vi "Ball Movement Graph with Air Resistance.vi"(0 "X Velocity Initial":dbl, 1 "Y Velocity Initial":dbl, 2 "Initial Angular Velocity":dbl, 3 "X Coordinate Initial":dbl, 4 "Y Coordinate Initial":dbl, 5 "Delta Time":dbl, 7 "milliseconds to wait":u32) -> (10 "Cross-Sectional Area":dbl, 12 "Drag Coefficient":dbl, 14 "Table":string[][](table), 15 "X of Y max":dbl, 16 "Y Max":dbl)   [LabVIEW 2013]
panel:
  out "Loop Count":i32
  out "Y Coordinate":dbl
  out "X Coordinate":dbl
  out "Angular Velocity":dbl
  out "Time":dbl
  out "Y Velocity":dbl
  out "X Velocity":dbl
  out "X Acceleration":dbl
  out "Y Acceleration":dbl
  # "This is in SI"
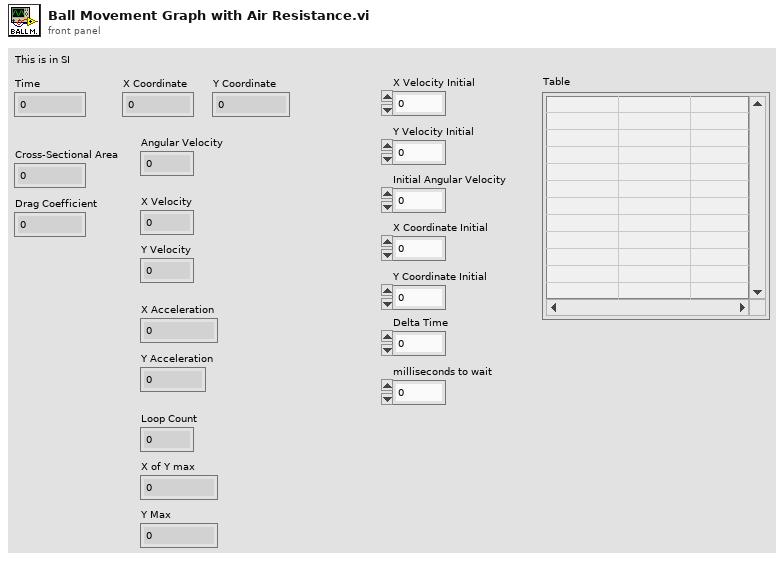
[diagram p1: front panel]
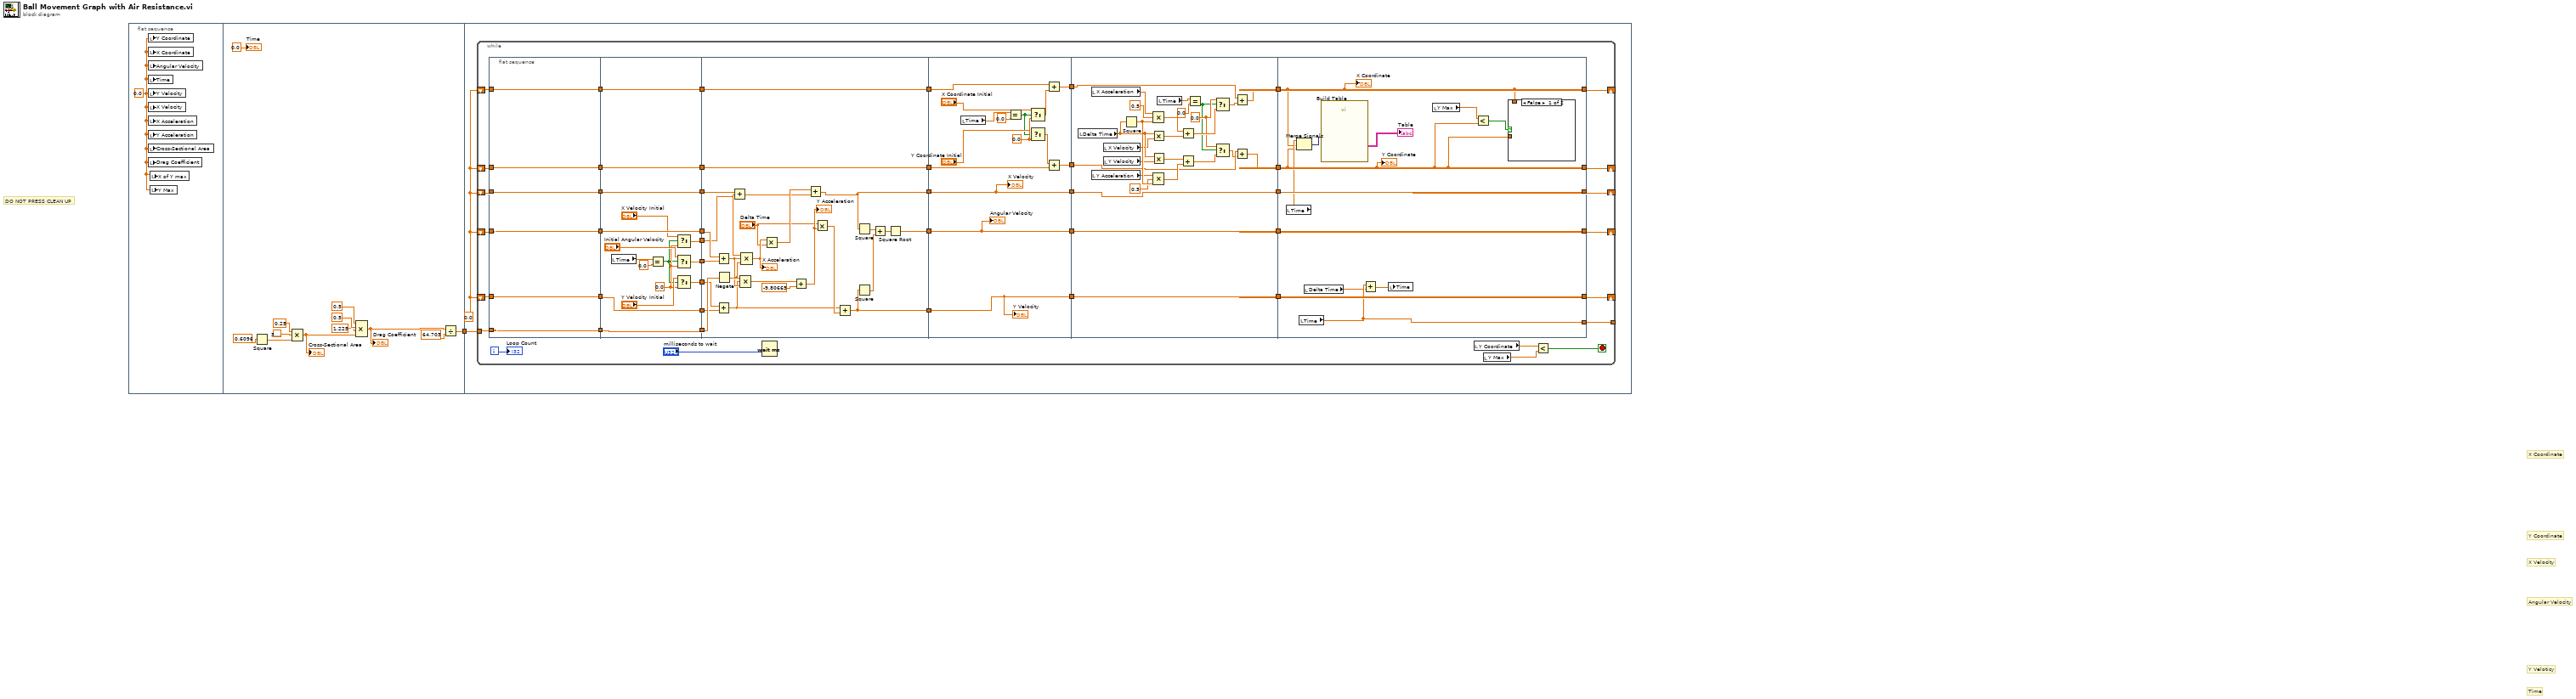
[diagram p0: block diagram]
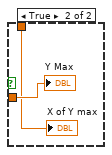
[diagram p2: hidden frame]
diagram:
  # "DO NOT PRESS CLEAN UP"
  # "Time"
  # "X Coordinate"
  # "Y Coordinate"
  # "Angular Velocity"
  # "X Velocity"
  # "Y Veloticy"
  n1 = flat-sequence {
    tunnel: [w6] -> w1
    tunnel: w1 -> [w16]
    frame #0 {
      w2 = 0.0
      n2 = local write "Y Coordinate"(w2) -> ()
      n3 = local write "X Coordinate"(w2) -> ()
      n4 = local write "Angular Velocity"(w2) -> ()
      n5 = local write "Time"(w2) -> ()
      n6 = local write "Y Velocity"(w2) -> ()
      n7 = local write "X Velocity"(w2) -> ()
      n8 = local write "X Acceleration"(w2) -> ()
      n9 = local write "Y Acceleration"(w2) -> ()
      n10 = local write "Cross-Sectional Area"(w2) -> ()
      n11 = local write "Drag Coefficient"(w2) -> ()
      n12 = local write "X of Y max"(w2) -> ()
      n13 = local write "Y Max"(w2) -> ()
    }
    frame #1 {
      n14 = Square(x=0.6096) -> (x^2=w4:dbl)
      n15 = Compound Arithmetic op=MULTIPLY(0.25 ("value"), 3.141592653589793, w4) -> (w3:dbl)
      "Cross-Sectional Area" <- w3
      n16 = Compound Arithmetic op=MULTIPLY(0.5 ("value"), 0.5 ("value"), 1.225 ("value"), w3) -> (w8:dbl)
      "Drag Coefficient" <- w8
      n17 = Divide(x=w8, y=64.703 ("x")) -> (x/y=w6:dbl)
      "Time" <- 0.0 ("Time")
    }
    frame #2 {
      w15 = 0.0
      n18 = while {
        tunnel: w16 -> [w57]
        shift-right: [w49] -> _
        shift-left: w15 -> [w22]
        shift-right: [w50] -> _
        shift-left: w15 -> [w58]
        shift-right: [w51] -> _
        shift-left: w15 -> [w19]
        shift-right: [w26] -> _
        shift-left: w15 -> [w20]
        shift-right: [w25] -> _
        shift-left: w15 -> [w21]
        tunnel: [w24] -> _
        i -> [w23]
        stop <- w27 stop-if-true
        n19 = flat-sequence {
          tunnel: w21 -> [w66]
          tunnel: w20 -> [w65]
          tunnel: w22 -> [w64]
          tunnel: w19 -> [w67]
          tunnel: w58 -> [w68]
          tunnel: w57 -> [w69]
          tunnel: [w69] -> w34
          tunnel: [w68] -> w33
          tunnel: [w67] -> w32
          tunnel: [w64] -> w31
          tunnel: [w65] -> w30
          tunnel: [w66] -> w29
          tunnel: [w85] -> w43
          tunnel: [w84] -> w42
          tunnel: [w70] -> w41
          tunnel: [w83] -> w40
          tunnel: [w82] -> w39
          tunnel: [w81] -> w38
          tunnel: [w80] -> w37
          tunnel: [w79] -> w36
          tunnel: [w78] -> w35
          tunnel: w34 -> [w85]
          tunnel: w33 -> [w84]
          tunnel: w32 -> [w70]
          tunnel: w31 -> [w83]
          tunnel: w30 -> [w82]
          tunnel: w29 -> [w81]
          tunnel: [w100] -> w63
          tunnel: [w110] -> w60
          tunnel: [w92] -> w56
          tunnel: [w91] -> w55
          tunnel: [w90] -> w52
          tunnel: w43 -> [w111]
          tunnel: w42 -> [w87]
          tunnel: w41 -> [w101]
          tunnel: w40 -> [w93]
          tunnel: w39 -> [w91]
          tunnel: w38 -> [w90]
          tunnel: w37 -> [w89]
          tunnel: w36 -> [w86]
          tunnel: w35 -> [w88]
          tunnel: w63 -> [w114]
          tunnel: [w114] -> w62
          tunnel: [w112] -> w61
          tunnel: w60 -> [w113]
          tunnel: [w113] -> w59
          tunnel: w56 -> [w112]
          tunnel: w55 -> [w115]
          tunnel: [w120] -> w54
          tunnel: [w119] -> w53
          tunnel: w52 -> [w116]
          tunnel: w62 -> [w153]
          tunnel: w61 -> [w151]
          tunnel: w59 -> [w152]
          tunnel: w54 -> [w140]
          tunnel: w53 -> [w137]
          tunnel: [w153] -> w48
          tunnel: [w151] -> w47
          tunnel: [w152] -> w46
          tunnel: [w139] -> w45
          tunnel: [w138] -> w44
          tunnel: [w156] -> w25
          tunnel: [w154] -> w26
          tunnel: [w163] -> w50
          tunnel: [w161] -> w49
          tunnel: [w162] -> w51
          tunnel: w48 -> [w162]
          tunnel: w47 -> [w161]
          tunnel: w46 -> [w163]
          tunnel: w45 -> [w154]
          tunnel: w44 -> [w156]
          tunnel: [w165] -> w24
          frame #0 {
          }
          frame #1 {
            w73 = 0.0
            n20 = local read "Time"() -> (w74:dbl)
            n21 = Equal?(x=w74, y=0.0) -> (x = y?=w72:bool)
            n22 = Select(t="X Velocity Initial", s=w72, f=w73) -> (s? t:f=w79:dbl)
            n23 = Select(t="Initial Angular Velocity", s=w72, f=w73) -> (s? t:f=w80:dbl)
            n24 = Select(t="Y Velocity Initial", s=w72, f=w73) -> (s? t:f=w78:dbl)
          }
          frame #2 {
            n25 = Add(x=w87, y=w89) -> (x+y=w106:dbl)
            n26 = Add(x=w88, y=w101) -> (x+y=w95:dbl)
            n27 = Negate(x=w111) -> (-x=w108:dbl)
            n28 = Add(x=w93, y=w86) -> (x+y=w102:dbl)
            n29 = Compound Arithmetic op=MULTIPLY(w108, w95, w106) -> (w96:dbl)
            n30 = Compound Arithmetic op=MULTIPLY(w102, w106, w108) -> (w97:dbl)
            "X Acceleration" <- w97
            n31 = Multiply(x=w97, y="Delta Time") -> (x*y=w109:dbl)
            n32 = Add(x=w96, y=-9.80665) -> (x+y=w98:dbl)
            "Y Acceleration" <- w98
            n33 = Add(x=w109, y=w102) -> (x+y=w92:dbl)
            n34 = Multiply(x="Delta Time", y=w98) -> (x*y=w99:dbl)
            n35 = Add(x=w95, y=w99) -> (x+y=w100:dbl)
            n36 = Square(x=w92) -> (x^2=w104:dbl)
            n37 = Square(x=w100) -> (x^2=w105:dbl)
            n38 = Add(x=w104, y=w105) -> (x+y=w103:dbl)
            n39 = Square Root(x=w103) -> (sqrt(x)=w110:dbl)
          }
          frame #3 {
            w123 = 0.0 ("f")
            n40 = local read "Time"() -> (w125:dbl)
            n41 = Equal?(x=w125, y=0.0) -> (x = y?=w117:bool)
            n42 = Select(t="X Coordinate Initial", s=w117, f=w123) -> (s? t:f=w121:dbl)
            n43 = Select(t="Y Coordinate Initial", s=w117, f=w123) -> (s? t:f=w118:dbl)
            n44 = Add(x=w115, y=w121) -> (x+y=w120:dbl)
            n45 = Add(x=w118, y=w116) -> (x+y=w119:dbl)
            "Angular Velocity" <- w113
            "X Velocity" <- w112
            "Y Velocity" <- w114
          }
          frame #4 {
            w130 = 0.0
            n46 = local read "Delta Time"() -> (w145:dbl)
            n47 = local read "X Acceleration"() -> (w147:dbl)
            n48 = local read "Y Acceleration"() -> (w146:dbl)
            n49 = local read "X Velocity"() -> (w135:dbl)
            n50 = local read "Y Velocity"() -> (w136:dbl)
            n51 = Square(x=w145) -> (x^2=w150:dbl)
            n52 = Multiply(x=w145, y=w135) -> (x*y=w144:dbl)
            n53 = Multiply(x=w145, y=w136) -> (x*y=w141:dbl)
            n54 = Compound Arithmetic op=MULTIPLY(w147, 0.5, w150) -> (w143:dbl)
            n55 = Compound Arithmetic op=MULTIPLY(w146, 0.5, w150) -> (w142:dbl)
            n56 = local read "Time"() -> (w134:dbl)
            n57 = Add(x=w143, y=w144) -> (x+y=w132:dbl)
            n58 = Add(x=w141, y=w142) -> (x+y=w131:dbl)
            n59 = Equal?(x=w134, y=0.0) -> (x = y?=w129:bool)
            n60 = Select(t=w130, s=w129, f=w132) -> (s? t:f=w127:dbl)
            n61 = Select(t=w130, s=w129, f=w131) -> (s? t:f=w128:dbl)
            n62 = Add(x=w140, y=w127) -> (x+y=w139:dbl)
            n63 = Add(x=w137, y=w128) -> (x+y=w138:dbl)
          }
          frame #5 {
            n64 = local read "Time"() -> (w160:dbl)
            n65 = Merge Signals(w160, w154, w156) -> (w158:dynamicdata)
            n66 = local read "Time"() -> (w165:dbl)
            n67 = local read "Delta Time"() -> (w164:dbl)
            n68 = call "Build Table"("Signals"=w158) -> ("Table"=→"Table":string[][])  [unwired: 4 in, 6 out]
            n69 = Add(x=w165, y=w164) -> (x+y=w166:dbl)
            n70 = local write "Time"(w166) -> ()
            n71 = local read "Y Max"() -> (w155:dbl)
            n72 = Less?(x=w155, y=w156) -> (x < y?=w157:bool)
            n73 = case shown="False" w157 {
              tunnel: w156 -> [_ w168]
              tunnel: w154 -> [_ w167]
              frame False {
              }
              frame True {
                "Y Max" <- w168
                "X of Y max" <- w167
              }
            }
            "Y Coordinate" <- w156
            "X Coordinate" <- w154
          }
        }
        n74 = Wait (ms)(milliseconds to wait="milliseconds to wait") -> ()  [unwired: 1 out]
        n75 = local read "Y Coordinate"() -> (w28:dbl)
        n76 = local read "Y Max"() -> (w17:dbl)
        n77 = Less?(x=w28, y=w17) -> (x < y?=w27:bool)
        "Loop Count" <- w23
      }
    }
  }
